vi "AutoDrive.vi"(4 "Timeout":u32=9900, 6 "Speed in":dbl=0.75, 7 "Mode":T2, 8 "error in (no error)":errorcluster, 9 "Angle in":dbl=180.0, 10 "Distance in":dbl=60.0, 11 "Command":T1) -> (0 "error out":errorcluster)   [LabVIEW 2013]
uses:
  AutoDriveModes.ctl
  AutoDriveCmds.ctl
  Position Typedef.ctl
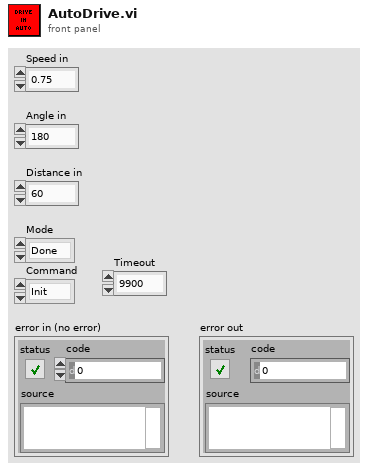
[diagram p1: front panel]
types:
  T1 = typedef "AutoDriveCmds.ctl" = enum16{"Init", "Set", "Run"}
  T2 = typedef "AutoDriveModes.ctl" = enum16{"Done", "Drive", "Turn"}
  T3 = typedef "Position Typedef.ctl" = cluster{"X":dbl, "Y":dbl, "Heading":dbl}
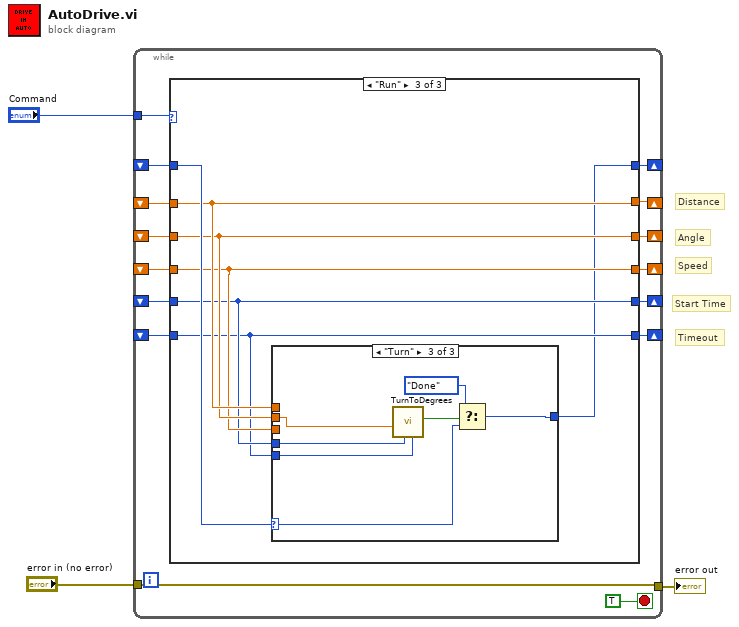
[diagram p0: block diagram]
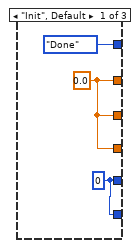
[diagram p2: hidden frame]
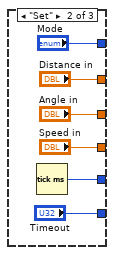
[diagram p3: hidden frame]
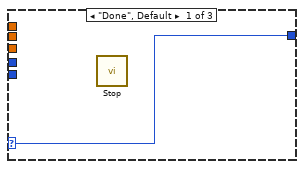
[diagram p4: hidden frame]
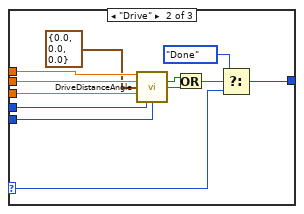
[diagram p5: hidden frame]
diagram:
  # "Timeout"
  # "Start Time"
  # "Speed"
  # "Angle"
  # "Distance"
  n1 = while {
    shift-right: [w16] -> _
    shift-left: _ -> [w17]
    shift-right: [w15] -> _
    shift-left: _ -> [w12]
    shift-right: [w14] -> _
    shift-left: _ -> [w11]
    shift-right: [w13] -> _
    shift-left: _ -> [w10]
    tunnel: "Command" -> [w9]
    tunnel: "error in (no error)" -> [w8]
    tunnel: [w8] -> w3
    shift-right: [w7] -> _
    shift-left: _ -> [w5]
    shift-right: [w6] -> _
    shift-left: _ -> [w4]
    stop <- TRUE stop-if-true
    n2 = case shown="\"Run\"" w9 {
      tunnel: w17 -> [_ _ w34]
      tunnel: [AutoDriveModes."Done" "Mode" w28] -> w16
      tunnel: [w20 "Distance in" w33] -> w15
      tunnel: [w20 "Angle in" w32] -> w14
      tunnel: [w20 "Speed in" w31] -> w13
      tunnel: w12 -> [_ _ w33]
      tunnel: w11 -> [_ _ w32]
      tunnel: w10 -> [_ _ w31]
      tunnel: [w19 w23 w30] -> w7
      tunnel: [w19 "Timeout" w29] -> w6
      tunnel: w5 -> [_ _ w30]
      tunnel: w4 -> [_ _ w29]
      frame "Init", Default {
        w19 = u32 0 ("millisecond timer value")
        w20 = 0.0 ("Distance 2")
      }
      frame "Set" {
        n3 = Tick Count (ms)() -> (millisecond timer value=w23:u32)
      }
      frame "Run" {
        n4 = case shown="\"Turn\"" w34 {
          selector: w34 -> [w35 w38 w50]
          tunnel: w33 -> [_ w47 _]
          tunnel: w32 -> [_ w46 w48]
          tunnel: w31 -> [_ w45 _]
          tunnel: w30 -> [_ w43 w54]
          tunnel: w29 -> [_ w42 w53]
          tunnel: [w35 w37 w52] -> w28
          frame "Done", Default {
            n5 = call "Stop.vi"() -> ()  [unwired: 12 in]
          }
          frame "Drive" {
            n6 = call "DriveDistanceAngle.vi"("Distance"=w47, "Angle"=w46, "Starting Position"=T3 {"X"=0.0, "Y"=0.0, "Heading"=0.0}, "Speed"=w45, "Start time"=w43, "Timeout (ms)"=w42) -> ("At Target"=w40:bool, "Timeout?"=w41:bool)  [unwired: 6 in, 2 out]
            n7 = Or(x=w40, y=w41) -> (x .or. y?=w39:bool)
            n8 = Select(t=AutoDriveModes."Done", s=w39, f=w38) -> (s? t:f=w37:T2)
          }
          frame "Turn" {
            n9 = call "TurnToDegrees.vi"("Timeout (ms)"=w53, "Start time"=w54, "Degrees"=w48) -> ("Done"=w51:bool)  [unwired: 6 in, 2 out]
            n10 = Select(t=AutoDriveModes."Done", s=w51, f=w50) -> (s? t:f=w52:T2)
          }
        }
      }
    }
  }
  "error out" <- w3
